vi "Serial Port Write.vi"(1 "string to write":string, 2 "port number":i32) -> (0 "error code":i32)   [LabVIEW 2020]
doc: "Writes the data in <B>string to write</B> to the serial port indicated in <B>port number</B>."
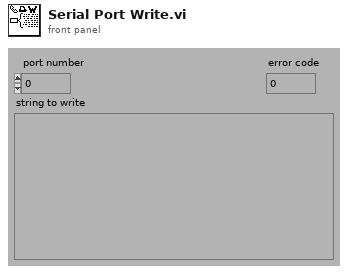
[diagram p1: front panel]
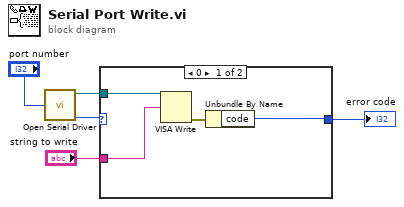
[diagram p0: block diagram]
diagram:
  n1 = call "Open Serial Driver.vi"("port number"="port number") -> ("input refnum"=w4:refnum<visa-resource-name>, "output error"=w3:i32)  [unwired: 2 out]
  n2 = case shown="0" w3 {
    selector: w3 -> [_ w10]
    tunnel: w4 -> [w9 _]
    tunnel: [w6 w10] -> w2
    tunnel: "string to write" -> [w8 _]
    frame 0 {
      n3 = VISA Write(VISA resource name=w9, write buffer=w8) -> (error out=w7:errorcluster)  [unwired: 1 in, 2 out]
      n4 = Unbundle By Name(w7) -> ("code"=w6:i32)
    }
    frame 1, Default {
    }
  }
  "error code" <- w2
